vi "IMS Stepper Control.vi"(2 "Point #":i32, 4 "Parameters":dbl[](array[numeric]) format="%.3e", 5 "Instrument Address":refnum<visa-resource-name>) -> (0 "Stop":bool, 1 "Data Out":dbl[](array[numeric]) format="%.2f")   [LabVIEW 2025]
doc: "Moves the stepper moter an appropriate amount based on the point number, step size and final position.\nScott Hannahs, NHMFL, March 1999\nAuthor: Scott Hannahs <sth@magnet.fsu.edu>\n\nThis software is licensed for use under the “MIT License\"\nCopyright (c) 2025 Scott Hannahs, sth@sth@magnet.sthnet.net\n\nPermission is hereby granted, free of charge, to any person obtaining a copy of this software and associated documentation files (the \"Software\"), to deal in the Software without restriction, including without limitation the rights to use, copy, modify, merge, publish, distribute, sublicense, and/or sell copies of the Software, and to permit persons to whom the Software is furnished to do so, subject to the following conditions: The above copyright notice and this permission notice shall be included in all copies or substantial portions of the Software.\n\nTHE SOFTWARE IS PROVIDED \"AS IS\", WITHOUT WARRANTY OF ANY KIND, EXPRESS OR IMPLIED, INCLUDING BUT NOT LIMITED TO THE WARRANTIES OF MERCHANTABILITY, FITNESS FOR A PARTICULAR PURPOSE AND NONINFRINGEMENT. IN NO EVENT SHALL THE AUTHORS OR COPYRIGHT HOLDERS BE LIABLE FOR ANY CLAIM, DAMAGES OR OTHER LIABILITY, WHETHER IN AN ACTION OF CONTRACT, TORT OR OTHERWISE, ARISING FROM, OUT OF OR IN CONNECTION WITH THE SOFTWARE OR THE USE OR OTHER DEALINGS IN THE SOFTWARE."
uses:
  Serial Support VISA.llb/Serial Actions.ctl
panel:
  out "Starting Position":dbl format="%.2f"
  # "Motor Number"
  # "Step Size"
  # "Final Position"
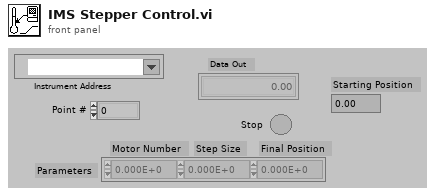
[diagram p1: front panel]
types:
  T1 = cluster{"Parameters[0]":dbl, "Parameters[1]":dbl, "Parameters[2]":dbl}
  T2 = typedef "Serial Actions.ctl" = enum16{"Init", "Break", "Clear Buffer", "Write", "Read", "N Bytes", "Lock", "Unlock", "Close"}
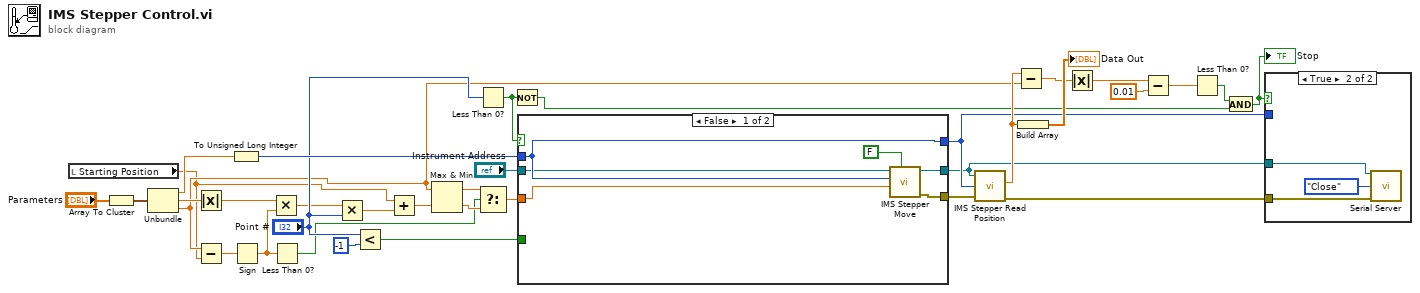
[diagram p0: block diagram]
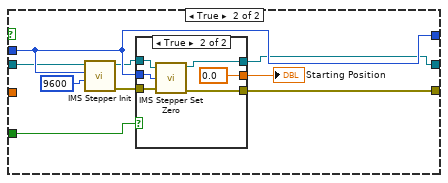
[diagram p3: hidden frame]
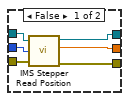
[diagram p4: hidden frame]
diagram:
  n1 = local read "Starting Position"() -> (w6:dbl)
  n2 = Array To Cluster(array="Parameters") -> (cluster=w34:T1)
  n3 = Unbundle(w34) -> ("Parameters[0]"=w31:dbl, "Parameters[1]"=w19:dbl, "Parameters[2]"=w12:dbl)
  n4 = Absolute Value(x=w19) -> (abs(x)=w17:dbl)
  n5 = Subtract(x=w12, y=w6) -> (x-y=w20:dbl)
  n6 = To Unsigned Long Integer(number=w31) -> (unsigned 32bit integer=w25:u32)
  n7 = Sign(1:w20) -> (0:w11:dbl)
  n8 = Multiply(x=w17, y=w11) -> (x*y=w18:dbl)
  n9 = Less Than 0?(x=w11) -> (x < 0?=w10:bool)
  n10 = Multiply(x=w18, y="Point #") -> (x*y=w33:dbl)
  n11 = Less?(x="Point #", y=-1) -> (x < y?=w22:bool)
  n12 = Add(x=w6, y=w33) -> (x+y=w16:dbl)
  n13 = Max & Min(x=w12, y=w16) -> (max(x,y)=w14:dbl, min(x,y)=w13:dbl)
  n14 = Less Than 0?(x="Point #") -> (x < 0?=w3:bool)
  n15 = Select(t=w14, s=w10, f=w13) -> (s? t:f=w15:dbl)
  n16 = Not(x=w3) -> (.not. x?=w2:bool)
  n17 = case shown="False" w3 {
    tunnel: "Instrument Address" -> [w37 w44]
    tunnel: [w36 w43] -> w26
    tunnel: w25 -> [w41 w46]
    tunnel: [w41 w46] -> w27
    tunnel: [w40 w49] -> w7
    tunnel: w22 -> [_ w48]
    tunnel: w15 -> [w39 _]
    frame False {
      n18 = call "IMS Stepper Move.vi"("Mode"=FALSE, "Distance"=w39, "Motor Number"=w41, "Instrument Address"=w37) -> ("error out"=w40:errorcluster, "Instrument Address Out"=w36:refnum<visa-resource-name>)  [unwired: 3 in]
    }
    frame True {
      n19 = call "IMS Stepper Init.vi"("Baud Rate"=u32 9600, "Motor Number"=w46, "Instrument Address"=w44) -> ("error out"=w45:errorcluster, "dup VISA Resource Name"=w42:refnum<visa-resource-name>)  [unwired: 2 in, 1 out]
      n20 = case shown="True" w48 {
        tunnel: w46 -> [w56 w62]
        tunnel: w42 -> [w55 w61]
        tunnel: [w54 w60] -> w49
        tunnel: [w53 0.0] -> w47
        tunnel: w45 -> [w52 w58]
        tunnel: [w51 w57] -> w43
        frame False {
          n21 = call "IMS Stepper Read Position.vi"("Instrument Address"=w55, "Motor Number"=w56, "error in (no error)"=w52) -> ("Instrument Address Out"=w51:refnum<visa-resource-name>, "Response"=w53:dbl, "error out"=w54:errorcluster)  [unwired: 1 in]
        }
        frame True {
          n22 = call "IMS Stepper Set Zero.vi"("Instrument Address"=w61, "Motor Number"=w62, "error in (no error)"=w58) -> ("Instrument Address Out"=w57:refnum<visa-resource-name>, "error out"=w60:errorcluster)  [unwired: 2 in]
        }
      }
      "Starting Position" <- w47
    }
  }
  n23 = call "IMS Stepper Read Position.vi"("Instrument Address"=w26, "Motor Number"=w27, "error in (no error)"=w7) -> ("Response"=w29:dbl, "error out"=w21:errorcluster)  [unwired: 1 in, 1 out]
  n24 = Subtract(x=w29, y=w12) -> (x-y=w28:dbl)
  n25 = Build Array(w29) -> (→"Data Out":dbl[])
  n26 = Absolute Value(x=w28) -> (abs(x)=w9:dbl)
  n27 = Subtract(x=w9, y=0.01) -> (x-y=w8:dbl)
  n28 = Less Than 0?(x=w8) -> (x < 0?=w4:bool)
  n29 = And(x=w4, y=w2) -> (x .and. y?=w5:bool)
  "Stop" <- w5
  n30 = case shown="True" w5 {
    tunnel: w27 -> [_ _]
    tunnel: w26 -> [_ w64]
    tunnel: w21 -> [_ w63]
    frame False {
    }
    frame True {
      n31 = call "Serial Server.vi"("VISA Resource Name"=w64, "Action"=Serial_Actions."Close", "error in (no error)"=w63) -> ()  [unwired: 8 in, 5 out]
    }
  }
